vi "p2.vi"() -> ()   [LabVIEW 2023, in "d18.lvlib"]
uses:
  d18.lvlib
  AOC/AOC.lvlib
  <vilib>/Analysis/NI_AAL_Geometry.lvlib
panel:
  out "XY Graph":cluster{dbl[], dbl[]}[](graph)
  in  "Example":string="R 6 (#70c710)\nD 5 (#0dc571)\nL 2 (#5713f0)\nD 2 (#d2c081)\nR 2 (#59c680)\nD 2 (#411b91)\nL 5 (#8ceee2)\nU 2 (#caa173)\nL 1 (#1b58a2)\nU 2 (#caa171)\nR 2 (#7807d2)\nU 3 (#a77fa3)\nL 2 (#015232)\nU 2 (#7a21e3)"
  in  "Example":bool
  out "Answer":u64
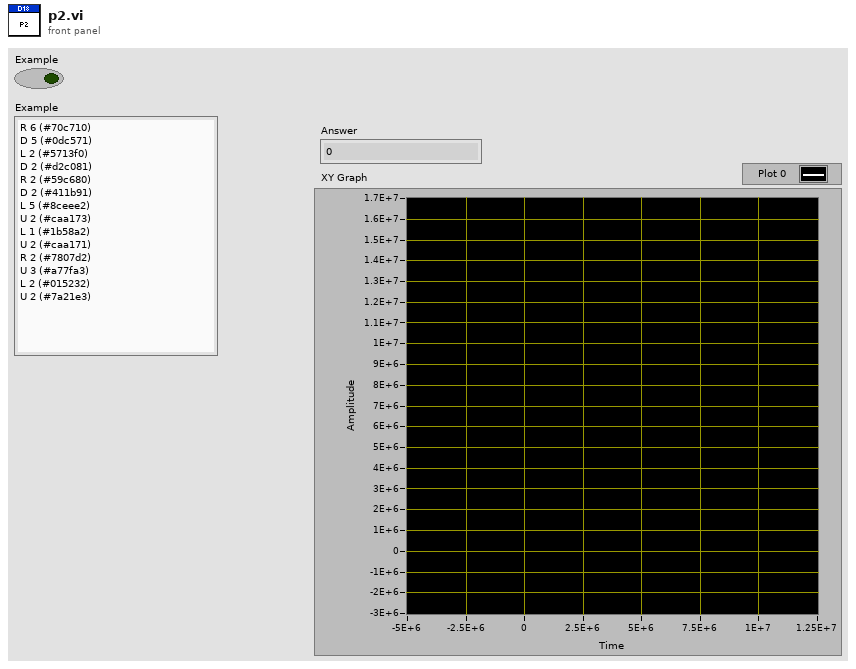
[diagram p1: front panel]
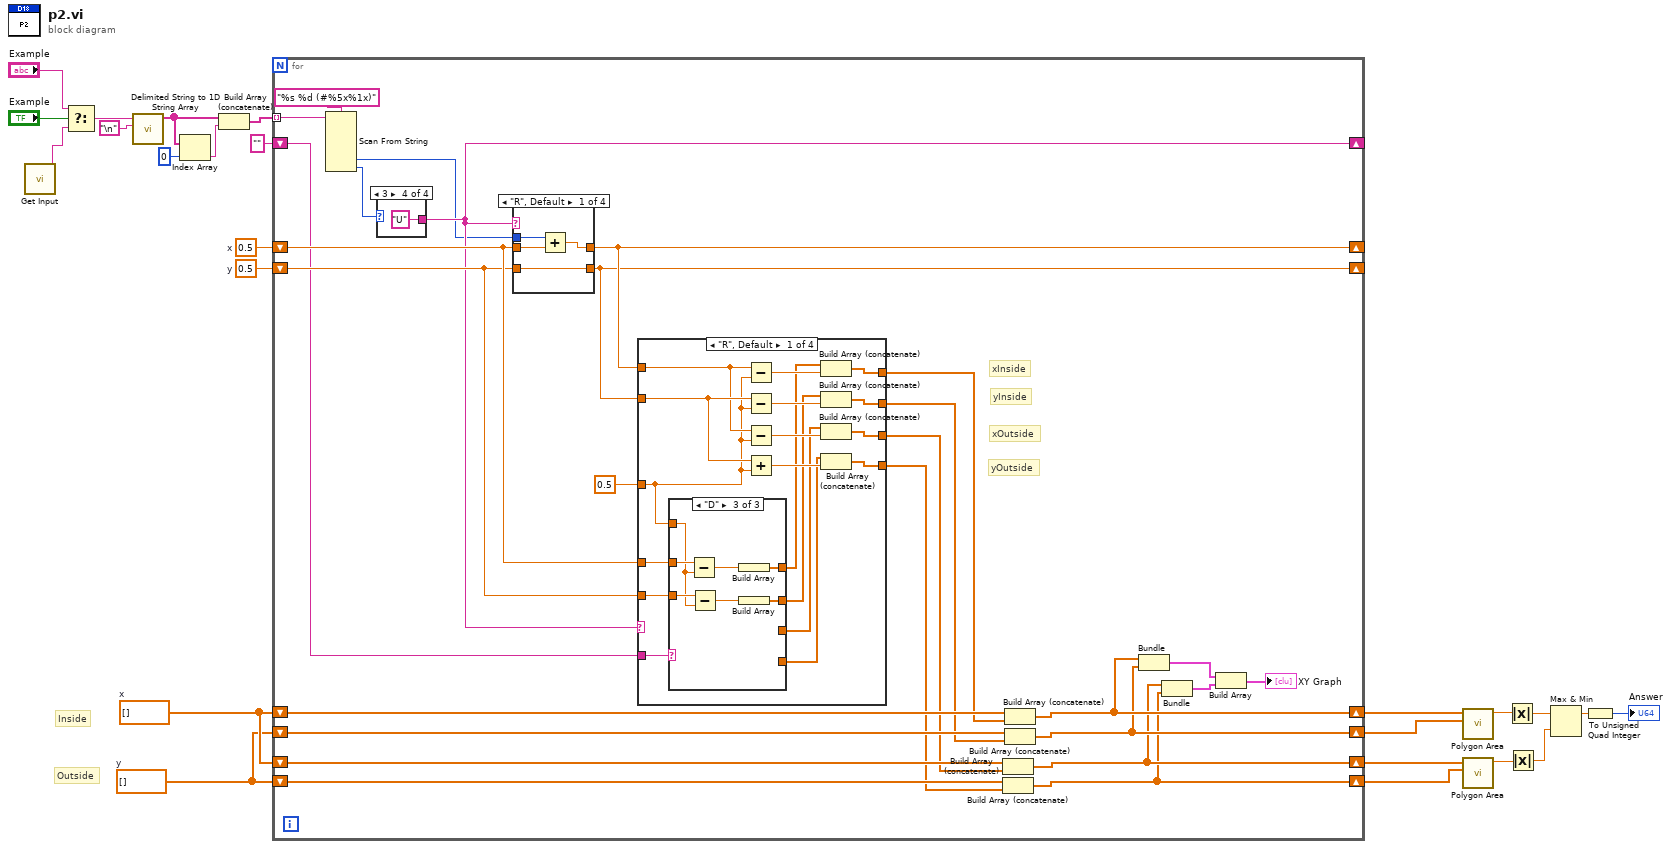
[diagram p0: block diagram]
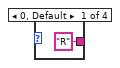
[diagram p2: hidden frame]
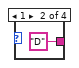
[diagram p3: hidden frame]
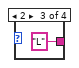
[diagram p4: hidden frame]
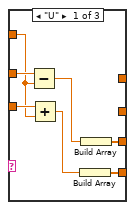
[diagram p5: hidden frame]
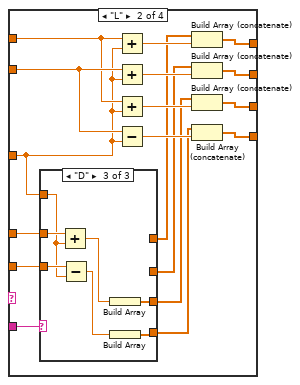
[diagram p7: hidden frame]
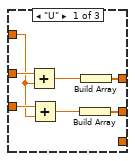
[diagram p8: hidden frame]
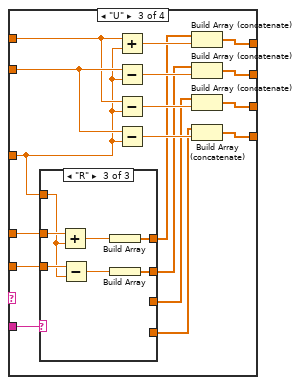
[diagram p10: hidden frame]
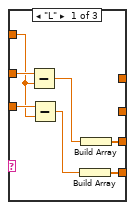
[diagram p11: hidden frame]
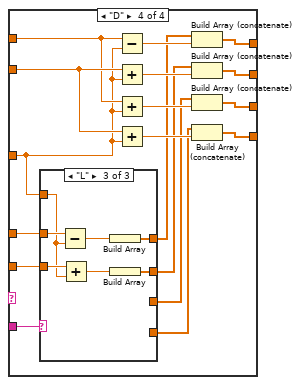
[diagram p13: hidden frame]
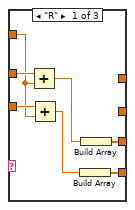
[diagram p14: hidden frame]
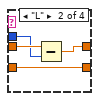
[diagram p16: hidden frame]
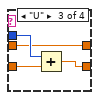
[diagram p17: hidden frame]
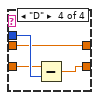
[diagram p18: hidden frame]
diagram:
  w18 = 0.5  # y
  w19 = 0.5  # x
  w14 = dbl[] []  # y
  w15 = dbl[] []  # x
  # "Outside"
  # "Inside"
  n1 = call "Get Input.vi"() -> ("Input"=w24:string)  [unwired: 11 in]
  n2 = Select(t="Example", s="Example", f=w24) -> (s? t:f=w23:string)
  n3 = call <vilib>:"Delimited String to 1D String Array.vi"("delimiter"="\n", "delimited string"=w23) -> ("string array"=w4:string[])  [unwired: 9 in]
  n4 = Index Array(array=w4, index=0) -> (element=w1:string)
  n5 = Build Array (concatenate)(w4, w1) -> (w2:string[])
  n6 = for {
    tunnel: w2 -> [w50] mode=indexing
    shift-right: [w34] -> w6
    shift-left: w15 -> [w48]
    shift-right: [w33] -> w5
    shift-left: w14 -> [w47]
    shift-right: [w43] -> _
    shift-left: w18 -> [w36]
    shift-right: [w44] -> _
    shift-left: w19 -> [w37]
    shift-right: [w32] -> w12
    shift-left: w15 -> [w46]
    shift-right: [w31] -> w11
    shift-left: w14 -> [w45]
    shift-right: [w26] -> _
    shift-left: "" -> [w35]
    # "yOutside"
    # "yInside"
    # "xOutside"
    # "xInside"
    n7 = Scan From String(format string="%s %d (#%5x%1x)", input string=w50) -> (output 3=w25:u32, output 4=w27:u32)  [unwired: 8 in, 3 out]
    n8 = case shown="3" w27 {
      tunnel: ["R" ("output 1") "D" ("output 1") "L" ("output 1") "U" ("output 1")] -> w26
      frame 0, Default {
      }
      frame 1 {
      }
      frame 2 {
      }
      frame 3 {
      }
    }
    n9 = case shown="\"R\", Default" w26 {
      tunnel: w37 -> [w186 w190 w191 w195]
      tunnel: w36 -> [w183 w187 w193 w197]
      tunnel: w25 -> [w185 w189 w194 w198]
      tunnel: [w184 w188 w191 w195] -> w44
      tunnel: [w183 w187 w192 w196] -> w43
      frame "R", Default {
        n10 = Add(x=w185, y=w186) -> (x+y=w184:dbl)
      }
      frame "L" {
        n11 = Subtract(x=w190, y=w189) -> (x-y=w188:dbl)
      }
      frame "U" {
        n12 = Add(x=w194, y=w193) -> (x+y=w192:dbl)
      }
      frame "D" {
        n13 = Subtract(x=w197, y=w198) -> (x-y=w196:dbl)
      }
    }
    n14 = case shown="\"R\", Default" w26 {
      tunnel: w44 -> [w65 w96 w128 w160]
      tunnel: [w72 w104 w136 w168] -> w42
      tunnel: [w71 w103 w134 w166] -> w41
      tunnel: [w70 w102 w133 w165] -> w40
      tunnel: [w69 w101 w132 w164] -> w39
      tunnel: w43 -> [w67 w99 w130 w162]
      tunnel: 0.5 ("y") -> [w59 w92 w123 w155]
      tunnel: w37 -> [w61 w95 w124 w156]
      tunnel: w36 -> [w60 w94 w125 w157]
      tunnel: w35 -> [w62 w93 w126 w158]
      frame "R", Default {
        n15 = case shown="\"D\"" w62 {
          tunnel: w61 -> [w79 _ w86]
          tunnel: w60 -> [w78 _ w85]
          tunnel: w59 -> [w77 _ w84]
          tunnel: [_ _ w82] -> w58
          tunnel: [_ _ w80] -> w57
          tunnel: [w73 _ _] -> w56
          tunnel: [w74 _ _] -> w55
          frame "U" {
            n16 = Subtract(x=w79, y=w77) -> (x-y=w76:dbl)
            n17 = Add(x=w78, y=w77) -> (x+y=w75:dbl)
            n18 = Build Array(w75) -> (w74:dbl[])
            n19 = Build Array(w76) -> (w73:dbl[])
          }
          frame "", Default {
          }
          frame "D" {
            n20 = Subtract(x=w86, y=w84) -> (x-y=w83:dbl)
            n21 = Subtract(x=w85, y=w84) -> (x-y=w81:dbl)
            n22 = Build Array(w83) -> (w82:dbl[])
            n23 = Build Array(w81) -> (w80:dbl[])
          }
        }
        n24 = Subtract(x=w65, y=w59) -> (x-y=w63:dbl)
        n25 = Subtract(x=w67, y=w59) -> (x-y=w68:dbl)
        n26 = Subtract(x=w65, y=w59) -> (x-y=w64:dbl)
        n27 = Add(x=w67, y=w59) -> (x+y=w66:dbl)
        n28 = Build Array (concatenate)(w58, w63) -> (w72:dbl[])
        n29 = Build Array (concatenate)(w57, w68) -> (w70:dbl[])
        n30 = Build Array (concatenate)(w56, w64) -> (w71:dbl[])
        n31 = Build Array (concatenate)(w55, w66) -> (w69:dbl[])
      }
      frame "L" {
        n32 = case shown="\"D\"" w93 {
          tunnel: w95 -> [w111 _ w118]
          tunnel: w94 -> [w110 _ w117]
          tunnel: w92 -> [w109 _ w116]
          tunnel: [w105 _ _] -> w90
          tunnel: [w106 _ _] -> w89
          tunnel: [_ _ w113] -> w88
          tunnel: [_ _ w112] -> w87
          frame "U" {
            n33 = Add(x=w111, y=w109) -> (x+y=w108:dbl)
            n34 = Add(x=w110, y=w109) -> (x+y=w107:dbl)
            n35 = Build Array(w107) -> (w106:dbl[])
            n36 = Build Array(w108) -> (w105:dbl[])
          }
          frame "", Default {
          }
          frame "D" {
            n37 = Add(x=w118, y=w116) -> (x+y=w115:dbl)
            n38 = Subtract(x=w117, y=w116) -> (x-y=w114:dbl)
            n39 = Build Array(w115) -> (w113:dbl[])
            n40 = Build Array(w114) -> (w112:dbl[])
          }
        }
        n41 = Add(x=w96, y=w92) -> (x+y=w91:dbl)
        n42 = Add(x=w99, y=w92) -> (x+y=w100:dbl)
        n43 = Add(x=w96, y=w92) -> (x+y=w97:dbl)
        n44 = Subtract(x=w99, y=w92) -> (x-y=w98:dbl)
        n45 = Build Array (concatenate)(w90, w91) -> (w104:dbl[])
        n46 = Build Array (concatenate)(w89, w100) -> (w102:dbl[])
        n47 = Build Array (concatenate)(w88, w97) -> (w103:dbl[])
        n48 = Build Array (concatenate)(w87, w98) -> (w101:dbl[])
      }
      frame "U" {
        n49 = case shown="\"R\"" w126 {
          tunnel: w124 -> [w143 _ w150]
          tunnel: w125 -> [w142 _ w149]
          tunnel: w123 -> [w141 _ w148]
          tunnel: [_ _ w146] -> w122
          tunnel: [_ _ w144] -> w121
          tunnel: [w137 _ _] -> w120
          tunnel: [w138 _ _] -> w119
          frame "L" {
            n50 = Subtract(x=w143, y=w141) -> (x-y=w140:dbl)
            n51 = Subtract(x=w142, y=w141) -> (x-y=w139:dbl)
            n52 = Build Array(w139) -> (w138:dbl[])
            n53 = Build Array(w140) -> (w137:dbl[])
          }
          frame "", Default {
          }
          frame "R" {
            n54 = Add(x=w150, y=w148) -> (x+y=w147:dbl)
            n55 = Subtract(x=w149, y=w148) -> (x-y=w145:dbl)
            n56 = Build Array(w147) -> (w146:dbl[])
            n57 = Build Array(w145) -> (w144:dbl[])
          }
        }
        n58 = Add(x=w128, y=w123) -> (x+y=w135:dbl)
        n59 = Subtract(x=w130, y=w123) -> (x-y=w131:dbl)
        n60 = Subtract(x=w128, y=w123) -> (x-y=w127:dbl)
        n61 = Subtract(x=w130, y=w123) -> (x-y=w129:dbl)
        n62 = Build Array (concatenate)(w122, w135) -> (w136:dbl[])
        n63 = Build Array (concatenate)(w121, w131) -> (w133:dbl[])
        n64 = Build Array (concatenate)(w120, w127) -> (w134:dbl[])
        n65 = Build Array (concatenate)(w119, w129) -> (w132:dbl[])
      }
      frame "D" {
        n66 = case shown="\"L\"" w158 {
          tunnel: w156 -> [w175 _ w182]
          tunnel: w157 -> [w174 _ w181]
          tunnel: w155 -> [w173 _ w180]
          tunnel: [_ _ w178] -> w154
          tunnel: [_ _ w176] -> w153
          tunnel: [w169 _ _] -> w152
          tunnel: [w170 _ _] -> w151
          frame "R" {
            n67 = Add(x=w175, y=w173) -> (x+y=w172:dbl)
            n68 = Add(x=w174, y=w173) -> (x+y=w171:dbl)
            n69 = Build Array(w171) -> (w170:dbl[])
            n70 = Build Array(w172) -> (w169:dbl[])
          }
          frame "", Default {
          }
          frame "L" {
            n71 = Subtract(x=w182, y=w180) -> (x-y=w179:dbl)
            n72 = Add(x=w181, y=w180) -> (x+y=w177:dbl)
            n73 = Build Array(w179) -> (w178:dbl[])
            n74 = Build Array(w177) -> (w176:dbl[])
          }
        }
        n75 = Subtract(x=w160, y=w155) -> (x-y=w167:dbl)
        n76 = Add(x=w162, y=w155) -> (x+y=w163:dbl)
        n77 = Add(x=w160, y=w155) -> (x+y=w159:dbl)
        n78 = Add(x=w162, y=w155) -> (x+y=w161:dbl)
        n79 = Build Array (concatenate)(w154, w167) -> (w168:dbl[])
        n80 = Build Array (concatenate)(w153, w163) -> (w165:dbl[])
        n81 = Build Array (concatenate)(w152, w159) -> (w166:dbl[])
        n82 = Build Array (concatenate)(w151, w161) -> (w164:dbl[])
      }
    }
    n83 = Build Array (concatenate)(w46, w41) -> (w32:dbl[])
    n84 = Build Array (concatenate)(w45, w39) -> (w31:dbl[])
    n85 = Build Array (concatenate)(w48, w42) -> (w34:dbl[])
    n86 = Build Array (concatenate)(w47, w40) -> (w33:dbl[])
    n87 = Bundle(w34, w33) -> (w30:cluster{dbl[], dbl[]})  [unwired: 1 in]
    n88 = Bundle(w32, w31) -> (w29:cluster{dbl[], dbl[]})  [unwired: 1 in]
    n89 = Build Array(w30, w29) -> (→"XY Graph":cluster{dbl[], dbl[]}[])
  }
  n90 = call <vilib>:"Polygon Area.vi"("Y"=w5, "X"=w6) -> ("signed area"=w17:dbl)  [unwired: 8 in, 1 out]
  n91 = call <vilib>:"Polygon Area.vi"("Y"=w11, "X"=w12) -> ("signed area"=w10:dbl)  [unwired: 8 in, 1 out]
  n92 = Absolute Value(x=w17) -> (abs(x)=w8:dbl)
  n93 = Absolute Value(x=w10) -> (abs(x)=w9:dbl)
  n94 = Max & Min(x=w8, y=w9) -> (max(x,y)=w7:dbl)  [unwired: 1 out]
  n95 = To Unsigned Quad Integer(1:w7) -> (0:→"Answer":u64)
